vi "rec_GapFreeDAQreplicates_v03.vi"(0 "AI task in":refnum<k21>, 1 "number of samples":i32=-1, 2 "controls array in":refnum<vi>[](array[refnum]), 3 "which clamp":enum16{"VClamp", "IClamp"}(ring), 4 "AO task in":refnum<k21>, 5 "error in":errorcluster, 9 "Duration (s)":dbl) -> (14 "AI task out":refnum<k21>, 15 "data out (pA or mV)":waveform(dbl)(graph), 16 "control array out":refnum<vi>[](array[refnum]), 18 "AO task out":refnum<k21>, 19 "error out":errorcluster)   [LabVIEW 2019]
uses:
  <vilib>/DAQmx/read.llb/DAQmx Read (Analog Wfm 1Chan NSamp).vi
  <vilib>/DAQmx/miscellaneous.llb/DAQmx Fill In Error Info.vi
  <resource>/objmgr/daqmx.rc
panel:
  out "AvailSampPerChan":u32
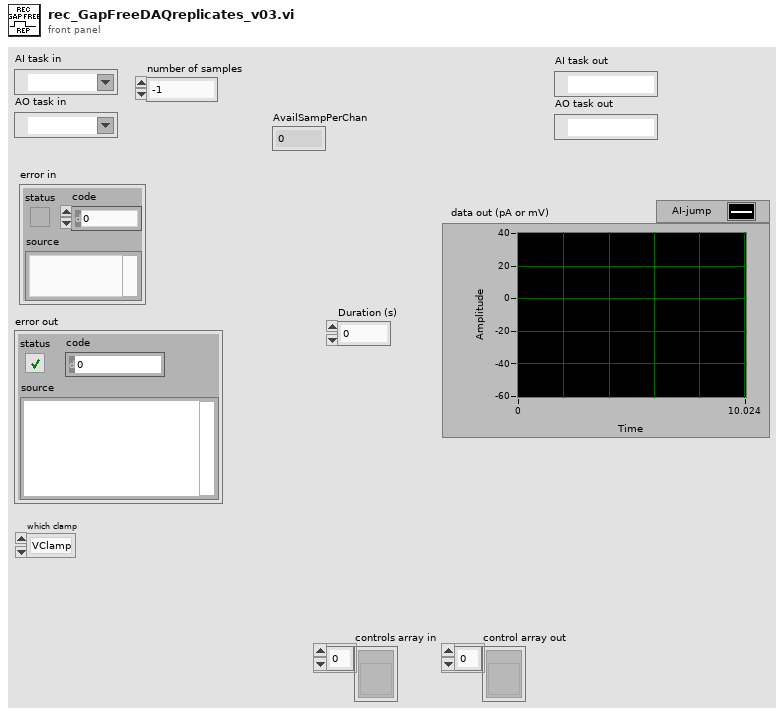
[diagram p1: front panel]
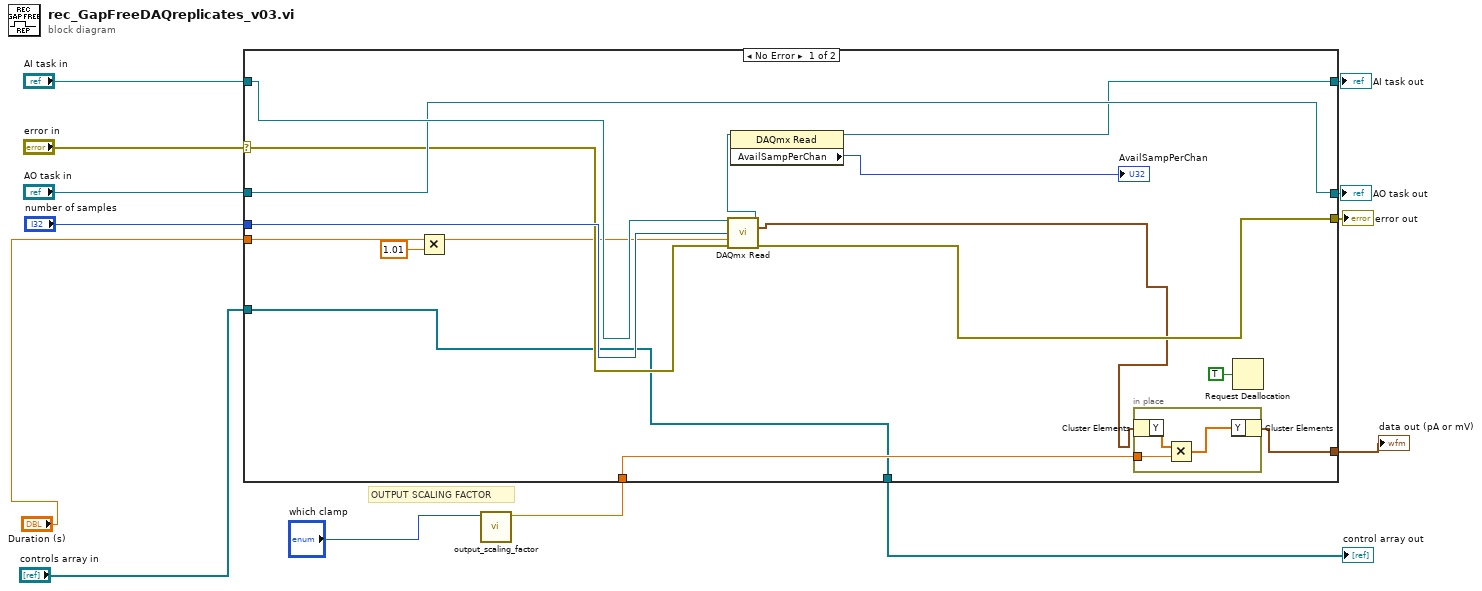
[diagram p0: block diagram]
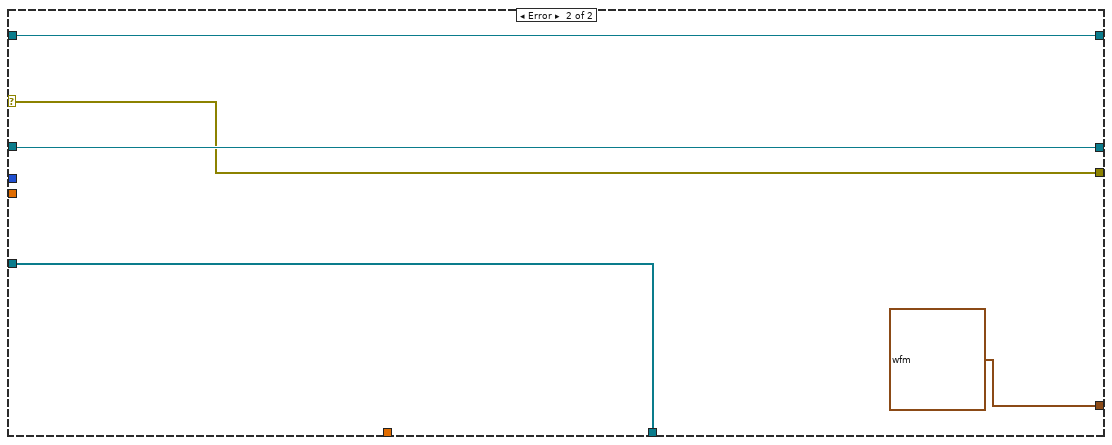
[diagram p2: hidden frame]
diagram:
  # "OUTPUT SCALING FACTOR"
  n1 = call "output_scaling_factor.vi"("which clamp"="which clamp") -> ("output scaling factor"=w7:dbl)  [unwired: 10 in]
  n2 = case shown="No Error" "error in" {
    selector: "error in" -> [w24 w35]
    tunnel: "AI task in" -> [w28 w37]
    tunnel: "AO task in" -> [w26 w36]
    tunnel: [w26 w36] -> w10
    tunnel: [w22 w37] -> w9
    tunnel: [w27 w35] -> w8
    tunnel: w7 -> [w29 _]
    tunnel: "number of samples" -> [w25 _]
    tunnel: "controls array in" -> [w23 w34]
    tunnel: [w23 w34] -> w4
    tunnel: "Duration (s)" -> [w20 _]
    tunnel: [w14 waveform(dbl) {"t0"=timestamp(0 s since 1904-01-01), "dt"=1.0, "Y"=[]}] -> w2
    frame No Error {
      n3 = Multiply(x=w20, y=1.01) -> (x*y=w19:dbl)
      n4 = call-poly <vilib>:"DAQmx Read.vi"("task/channels in"=w28, "number of samples per channel"=w25, "timeout"=w19, "error in"=w24) -> ("task out"=w16:refnum<k21>, "data"=w15:waveform(dbl), "error out"=w27:errorcluster)  [unwired: 9 in]
      n5 = property class="DAQmx Read"(reference=w16) -> (reference out=w22:refnum<k21>, "AvailSampPerChan"=→"AvailSampPerChan":u32)  [unwired: 1 in, 1 out]
      n6 = in-place {
        in-place-border: w29 -> [w32]
        n7 = in-place-cluster #1(w15) -> ("Y"=w30:dbl[])
        n8 = Multiply(x=w30, y=w32) -> (x*y=w31:dbl[])
        n9 = in-place-cluster #1("Y"=w31) -> (w14:waveform(dbl))
      }
      n10 = Request Deallocation(TRUE ("flag")) -> ()
    }
    frame Error {
    }
  }
  "AI task out" <- w9
  "AO task out" <- w10
  "error out" <- w8
  "control array out" <- w4
  "data out (pA or mV)" <- w2
